vi "实验第三题.vi"() -> ()   [LabVIEW 2018]
uses:
  <vilib>/Analysis/2dsp.llb/Real FFT.vi
  <vilib>/Analysis/1siggen.llb/Ramp Pattern by Samples.vi
  <vilib>/Analysis/NI_AALBase.lvlib
  <vilib>/Analysis/NI_AALPro.lvlib
panel:
  in  "停止 2":bool
  out "频域图":dbl[](graph)
  out "带噪声的波形":dbl[](graph)
  out "原波形":dbl[](graph)
  out "XY图 2":cluster{"square wave":dbl[], dbl[]}(graph)
  in  "停止":bool
  in  "相位":dbl(slide) scale=0.0..360.0
  in  "频率":dbl(slide) scale=0.0..5.0
  out "XY图":cluster{"sine wave":dbl[], "sine wave":dbl[]}(graph)
  # "第一题"
  # "第二题"
  # "第三题"
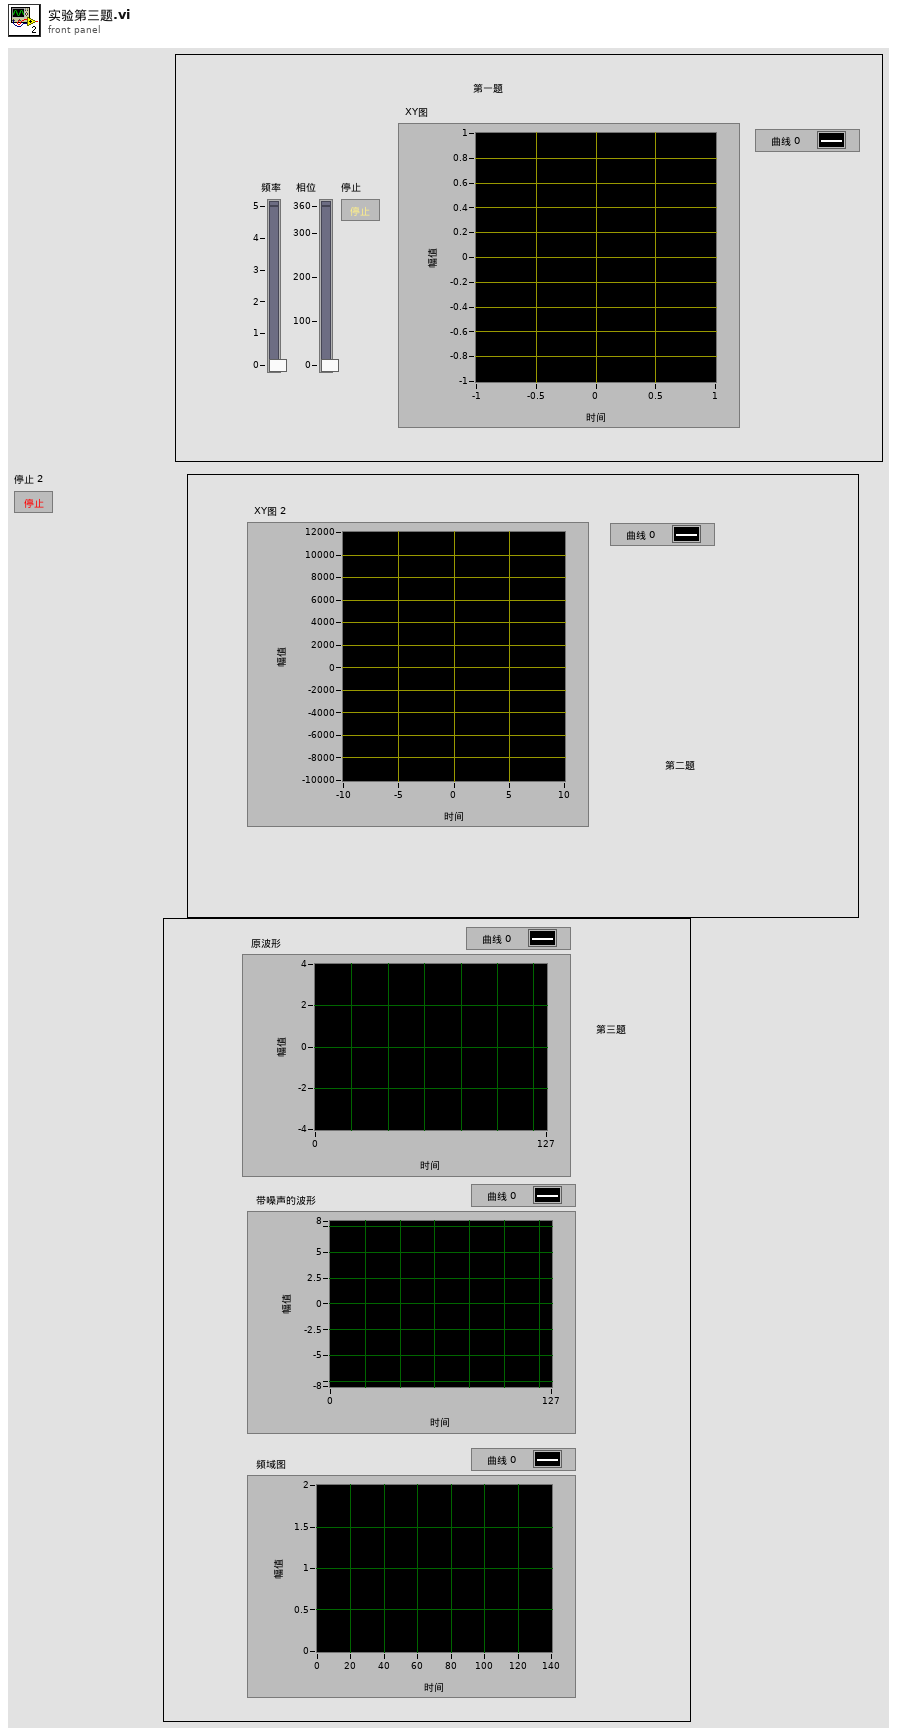
[diagram p1: front panel]
types:
  T1 = cluster{"Ramp Pattern":dbl[], "Ramp Pattern":dbl[]}
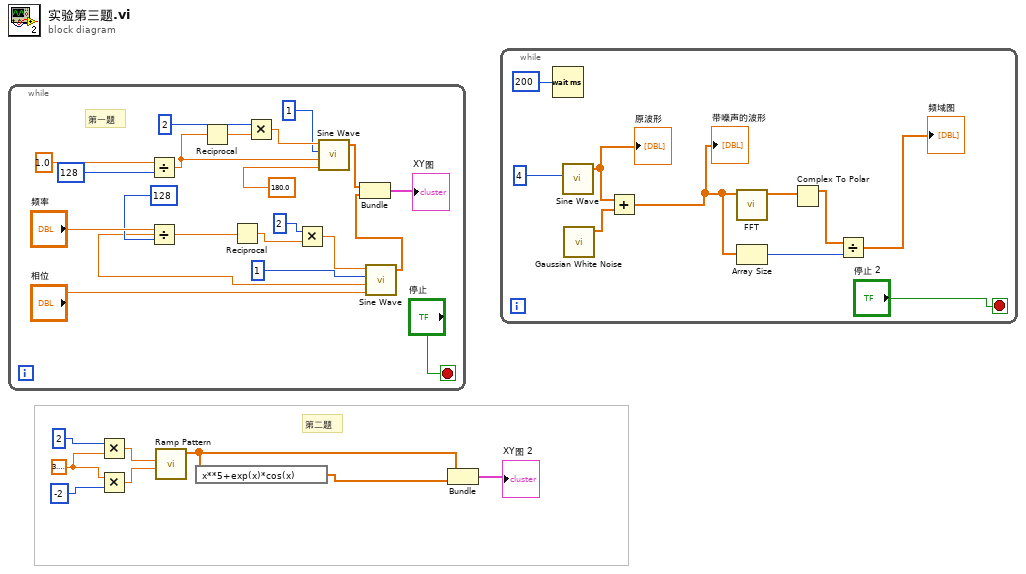
[diagram p0: block diagram]
diagram:
  w7 = 3.141592653589793
  # "第二题"
  n1 = while {
    stop <- "停止" stop-if-true
    # "第一题"
    n2 = Divide(x=1.0, y=128) -> (x/y=w22:dbl)
    n3 = Divide(x="频率", y=128) -> (x/y=w14:dbl)
    n4 = Reciprocal(x=w22) -> (1/x=w26:dbl)
    n5 = Reciprocal(x=w14) -> (1/x=w18:dbl)
    n6 = Multiply(x=2, y=w26) -> (x*y=w24:dbl)
    n7 = Multiply(x=2, y=w18) -> (x*y=w16:dbl)
    n8 = call <vilib>:"Sine Wave.vi"("samples"=w24, "amplitude"=1, "frequency"=w22, "phase in"=180.0) -> ("sine wave"=w11:dbl[])  [unwired: 1 in, 2 out]
    n9 = call <vilib>:"Sine Wave.vi"("samples"=w16, "amplitude"=1, "frequency"=w14, "phase in"="相位") -> ("sine wave"=w12:dbl[])  [unwired: 1 in, 2 out]
    n10 = Bundle("sine wave"=w11, "sine wave"=w12) -> (→"XY图":cluster{"sine wave":dbl[], "sine wave":dbl[]})  [unwired: 1 in]
  }
  n11 = Multiply(x=2, y=w7) -> (x*y=w5:dbl)
  n12 = Multiply(x=w7, y=-2) -> (x*y=w4:dbl)
  n13 = call-poly <vilib>:"Ramp Pattern.vi"("start"=w4, "end"=w5) -> ("Ramp Pattern"=w3:dbl[])  [unwired: 8 in, 1 out]
  n14 = expression code="x**5+exp(x)*cos(x)"(w3) -> (w2:dbl[])
  n15 = Bundle("Ramp Pattern"=w3, "Ramp Pattern"=w2) -> (→"XY图 2":T1)  [unwired: 1 in]
  n16 = while {
    stop <- "停止 2" stop-if-true
    n17 = Wait (ms)(milliseconds to wait=200) -> ()  [unwired: 1 out]
    n18 = call <vilib>:"Sine Wave.vi"("amplitude"=4) -> ("sine wave"=w36:dbl[])  [unwired: 4 in, 2 out]
    "原波形" <- w36
    n19 = call <vilib>:"Gaussian White Noise.vi"() -> ("Gaussian noise pattern"=w35:dbl[])  [unwired: 10 in, 1 out]
    n20 = Add(x=w36, y=w35) -> (x+y=w33:dbl[])
    "带噪声的波形" <- w33
    n21 = call-poly <vilib>:"FFT.vi"("X"=w33) -> ("FFT {X}"=w34:cdb[])  [unwired: 9 in, 1 out]
    n22 = Array Size(array=w33) -> (size(s)=w31:i32)
    n23 = Complex To Polar(r * e^(i*theta)=w34) -> (r=w32:dbl[])  [unwired: 1 out]
    n24 = Divide(x=w32, y=w31) -> (x/y=→"频域图":dbl[])
  }
